vi "data_waypoint_ref.vi"() -> ()   [LabVIEW 2018] (continued)
"Y"=530209.4196220397}, {"X"=175331.62295978758, "Y"=530209.4709902672}, {"X"=175331.66061267612, "Y"=530209.5217040731}, {"X"=175331.69814321943, "Y"=530209.5723827237}, {"X"=175331.73536540987, "Y"=530209.6233275409}, {"X"=175331.77258882776, "Y"=530209.6746885533}, {"X"=175331.80997591818, "Y"=530209.7262832607}, {"X"=175331.8481199299, "Y"=530209.7774340136}, {"X"=175331.88623244286, "Y"=530209.8287158216}, {"X"=175331.9241847472, "Y"=530209.8794387324}, {"X"=175331.96143662307, "Y"=530209.9299384085}, {"X"=175331.99790744064, "Y"=530209.9799065489}, {"X"=175332.03363035072, "Y"=530210.0303718917}, {"X"=175332.07052518567, "Y"=530210.0802477727}, {"X"=175332.10833857156, "Y"=530210.1304217139}, {"X"=175332.14653489395, "Y"=530210.1818897336}, {"X"=175332.1846024039, "Y"=530210.2341328121}, {"X"=175332.22300738035, "Y"=530210.2869697822}, {"X"=175332.2621362657, "Y"=530210.339582644}, {"X"=175332.30199405577, "Y"=530210.3918626182}, {"X"=175332.34141600237, "Y"=530210.4441305593}, {"X"=175332.38041804795, "Y"=530210.4963853122}, {"X"=175332.4185211116, "Y"=530210.5486704636}, {"X"=175332.45682697443, "Y"=530210.5997386106}, {"X"=175332.49514308042, "Y"=530210.6506768743}, {"X"=175332.53412157384, "Y"=530210.7006542655}, {"X"=175332.57272378285, "Y"=530210.7512909137}, {"X"=175332.61101197888, "Y"=530210.8029773051}, {"X"=175332.64921056182, "Y"=530210.8558148851}, {"X"=175332.68851538797, "Y"=530210.9095182215}, {"X"=175332.72771294997, "Y"=530210.9640942254}, {"X"=175332.76750234602, "Y"=530211.0190136484}, {"X"=175332.80752506072, "Y"=530211.0731554804}, {"X"=175332.84765670967, "Y"=530211.1269895624}, {"X"=175332.88795444716, "Y"=530211.1803758806}, {"X"=175332.92839109115, "Y"=530211.234007068}, {"X"=175332.96848531367, "Y"=530211.2886669956}, {"X"=175333.0089040344, "Y"=530211.3437299544}, {"X"=175333.0491415058, "Y"=530211.3989066537}, {"X"=175333.08910233053, "Y"=530211.4539887221}, {"X"=175333.1285585995, "Y"=530211.5088869324}, {"X"=175333.16815412405, "Y"=530211.5626471259}, {"X"=175333.20753422027, "Y"=530211.6163446938}, {"X"=175333.2473421582, "Y"=530211.6697457767}, {"X"=175333.28705198405, "Y"=530211.724119386}, {"X"=175333.3265540142, "Y"=530211.779216127}, {"X"=175333.3660775373, "Y"=530211.8349931492}, {"X"=175333.40622949848, "Y"=530211.8900102822}, {"X"=175333.44650034822, "Y"=530211.9444932247}, {"X"=175333.48723672854, "Y"=530211.9985430562}, {"X"=175333.52736064664, "Y"=530212.0530630564}, {"X"=175333.56740341955, "Y"=530212.1080017141}, {"X"=175333.6077093309, "Y"=530212.1626599086}, {"X"=175333.64857199727, "Y"=530212.2168813988}, {"X"=175333.68922026566, "Y"=530212.2707905404}, {"X"=175333.72890749428, "Y"=530212.3247113958}, {"X"=175333.76778450757, "Y"=530212.3784270975}, {"X"=175333.80736747183, "Y"=530212.4321351693}, {"X"=175333.84828877196, "Y"=530212.4858159842}, {"X"=175333.88984022452, "Y"=530212.539917797}, {"X"=175333.93109660895, "Y"=530212.5948872815}, {"X"=175333.97284515807, "Y"=530212.6497432184}, {"X"=175334.0142686215, "Y"=530212.7046001133}, {"X"=175334.05544437704, "Y"=530212.7586608616}, {"X"=175334.0959890387, "Y"=530212.8128810698}, {"X"=175334.13627522383, "Y"=530212.8671608662}, {"X"=175334.17651603464, "Y"=530212.9222742985}, {"X"=175334.2177644458, "Y"=530212.9772438075}, {"X"=175334.25957639978, "Y"=530213.0322760266}, {"X"=175334.30213095952, "Y"=530213.0865147257}, {"X"=175334.34455506905, "Y"=530213.1406738986}, {"X"=175334.38594238626, "Y"=530213.195288953}, {"X"=175334.42704816477, "Y"=530213.2499525625}, {"X"=175334.46824282644, "Y"=530213.3047191269}, {"X"=175334.50961381703, "Y"=530213.3595051488}, {"X"=175334.55108627415, "Y"=530213.4141565791}, {"X"=175334.59266786097, "Y"=530213.4679675244}, {"X"=175334.63399788298, "Y"=530213.5211776675}, {"X"=175334.6750819692, "Y"=530213.573293105}, {"X"=175334.71570326976, "Y"=530213.6252711763}, {"X"=175334.75589895574, "Y"=530213.6780007676}, {"X"=175334.79658751158, "Y"=530213.7311584209}, {"X"=175334.83711118187, "Y"=530213.7854730334}, {"X"=175334.87751620755, "Y"=530213.8401054167}, {"X"=175334.9179042401, "Y"=530213.894081924}, {"X"=175334.95911596806, "Y"=530213.9465288344}, {"X"=175334.99991220928, "Y"=530213.9986573323}, {"X"=175335.04026648914, "Y"=530214.050201127}, {"X"=175335.08012203232, "Y"=530214.1026320615}, {"X"=175335.12058568108, "Y"=530214.1555184657}, {"X"=175335.16164489972, "Y"=530214.2088137578}, {"X"=175335.2026623043, "Y"=530214.2629493396}, {"X"=175335.24292566493, "Y"=530214.317904002}, {"X"=175335.2838600399, "Y"=530214.3724194007}, {"X"=175335.32589039847, "Y"=530214.4264254693}, {"X"=175335.36913003057, "Y"=530214.4801915719}, {"X"=175335.4125249086, "Y"=530214.5343367882}, {"X"=175335.45555095756, "Y"=530214.5889669928}, {"X"=175335.49830331592, "Y"=530214.6433027806}, {"X"=175335.54073540578, "Y"=530214.6974685959}, {"X"=175335.58196774634, "Y"=530214.7521007617}, {"X"=175335.62354322325, "Y"=530214.8059483555}, {"X"=175335.66565024323, "Y"=530214.8586179304}, {"X"=175335.70747625933, "Y"=530214.9106157594}, {"X"=175335.7480881228, "Y"=530214.963002292}, {"X"=175335.7885573149, "Y"=530215.0144669515}, {"X"=175335.82880391076, "Y"=530215.0658434787}, {"X"=175335.86905572907, "Y"=530215.1162866012}, {"X"=175335.909482951, "Y"=530215.1667380838}, {"X"=175335.95024341732, "Y"=530215.2175526178}, {"X"=175335.9909282017, "Y"=530215.2700366036}, {"X"=175336.03225353497, "Y"=530215.3231646375}, {"X"=175336.0742294917, "Y"=530215.3758479197}, {"X"=175336.1162228887, "Y"=530215.4281371495}, {"X"=175336.15780792251, "Y"=530215.480420926}, {"X"=175336.198753351, "Y"=530215.5338830402}, {"X"=175336.2400447598, "Y"=530215.5884240265}, {"X"=175336.28280096015, "Y"=530215.6431649067}, {"X"=175336.32627274963, "Y"=530215.697862611}, {"X"=175336.3695396637, "Y"=530215.7518728063}, {"X"=175336.41189431006, "Y"=530215.8050133444}, {"X"=175336.4530581296, "Y"=530215.857140764}, {"X"=175336.4923324384, "Y"=530215.9083226097}, {"X"=175336.53024073623, "Y"=530215.9582587824}, {"X"=175336.56758054454, "Y"=530216.0079569012}, {"X"=175336.60624975662, "Y"=530216.0567010613}, {"X"=175336.64522401133, "Y"=530216.1052567544}, {"X"=175336.68329837156, "Y"=530216.1538350807}, {"X"=175336.72042406868, "Y"=530216.2021165418}, {"X"=175336.75789178454, "Y"=530216.2498342964}, {"X"=175336.79601195845, "Y"=530216.2977277045}, {"X"=175336.83490120104, "Y"=530216.3474945049}, {"X"=175336.8747391946, "Y"=530216.3987878956}, {"X"=175336.9155644031, "Y"=530216.4511349584}, {"X"=175336.9565872925, "Y"=530216.5038343738}, {"X"=175336.99702923294, "Y"=530216.5562757964}, {"X"=175337.03653662247, "Y"=530216.608701107}, {"X"=175337.07562676386, "Y"=530216.6599112444}, {"X"=175337.11431845836, "Y"=530216.7105731766}, {"X"=175337.15316399393, "Y"=530216.7608384356}, {"X"=175337.19213873718, "Y"=530216.8122653349}, {"X"=175337.232309873, "Y"=530216.8641903627}, {"X"=175337.27302243776, "Y"=530216.9167896998}, {"X"=175337.31390302093, "Y"=530216.9698935254}, {"X"=175337.3542175054, "Y"=530217.0235705986}, {"X"=175337.39383505605, "Y"=530217.0782097556}, {"X"=175337.43345427106, "Y"=530217.1331130541}, {"X"=175337.4731671136, "Y"=530217.1885266124}, {"X"=175337.51269825146, "Y"=530217.2435999815}, {"X"=175337.55194491986, "Y"=530217.2977274793}, {"X"=175337.59038441366, "Y"=530217.3505776902}, {"X"=175337.62842923752, "Y"=530217.40235916}, {"X"=175337.6661001939, "Y"=530217.4535179922}, {"X"=175337.70416076016, "Y"=530217.5037300759}, {"X"=175337.7420038972, "Y"=530217.5544022826}, {"X"=175337.7794317696, "Y"=530217.6051323175}, {"X"=175337.81701866104, "Y"=530217.6563202547}, {"X"=175337.8544032769, "Y"=530217.708001567}, {"X"=175337.8925377935, "Y"=530217.7595608027}, {"X"=175337.93128742423, "Y"=530217.8109495258}, {"X"=175337.9695507337, "Y"=530217.8629301275}, {"X"=175338.0082516581, "Y"=530217.9152235296}, {"X"=175338.04761985684, "Y"=530217.967611521}, {"X"=175338.08728319546, "Y"=530218.0209597816}, {"X"=175338.1271335317, "Y"=530218.0749423284}, {"X"=175338.16702309356, "Y"=530218.1290091096}, {"X"=175338.20661768012, "Y"=530218.1830734315}, {"X"=175338.2461740608, "Y"=530218.2367982493}, {"X"=175338.28507050654, "Y"=530218.2905139152}, {"X"=175338.32402685797, "Y"=530218.3435179845}, {"X"=175338.3628983841, "Y"=530218.3962936742}, {"X"=175338.40248170623, "Y"=530218.4477409829}, {"X"=175338.44199884526, "Y"=530218.4989731741}, {"X"=175338.4810465143, "Y"=530218.5499037582}, {"X"=175338.51934318643, "Y"=530218.600885391}, {"X"=175338.55710943416, "Y"=530218.6522204147}, {"X"=175338.5948762553, "Y"=530218.7037507715}, {"X"=175338.6338252904, "Y"=530218.7548769822}, {"X"=175338.6739002579, "Y"=530218.8060364973}, {"X"=175338.71384854216, "Y"=530218.8583928163}, {"X"=175338.753222827, "Y"=530218.9113457106}, {"X"=175338.792356318, "Y"=530218.9646467023}, {"X"=175338.8311580059, "Y"=530219.01837153}, {"X"=175338.87071642242, "Y"=530219.0715880294}, {"X"=175338.91075334582, "Y"=530219.1254668134}, {"X"=175338.95190623117, "Y"=530219.1793034604}, {"X"=175338.99320496703, "Y"=530219.2336380056}, {"X"=175339.03450596903, "Y"=530219.2878393602}, {"X"=175339.07593600373, "Y"=530219.3419426669}, {"X"=175339.1173234146, "Y"=530219.3954090409}, {"X"=175339.15756587937, "Y"=530219.4490019855}, {"X"=175339.196607049, "Y"=530219.5022366615}, {"X"=175339.23502417348, "Y"=530219.5550181346}, {"X"=175339.27417272714, "Y"=530219.6071215451}, {"X"=175339.31415161595, "Y"=530219.6584433867}, {"X"=175339.35397403524, "Y"=530219.7095736838}, {"X"=175339.3928394618, "Y"=530219.7608854916}, {"X"=175339.43153280398, "Y"=530219.8121156775}, {"X"=175339.4711378264, "Y"=530219.8631167639}, {"X"=175339.5113195704, "Y"=530219.9153447627}, {"X"=175339.5514793716, "Y"=530219.968542844}, {"X"=175339.59169131416, "Y"=530220.0223001395}, {"X"=175339.63130955625, "Y"=530220.077183476}, {"X"=175339.6713096225, "Y"=530220.1317837801}, {"X"=175339.71162398445, "Y"=530220.1860302234}, {"X"=175339.75238126508, "Y"=530220.2396849147}, {"X"=175339.79291413393, "Y"=530220.2938363759}, {"X"=175339.8341795131, "Y"=530220.3476771363}, {"X"=175339.87538622756, "Y"=530220.4017489201}, {"X"=175339.91570330068, "Y"=530220.4557134501}, {"X"=175339.95501255686, "Y"=530220.5094489943}, {"X"=175339.99378179503, "Y"=530220.5623881428}, {"X"=175340.032220397, "Y"=530220.614045269}, {"X"=175340.0706813909, "Y"=530220.6642850373}, {"X"=175340.1095277134, "Y"=530220.7136280148}, {"X"=175340.1483784491, "Y"=530220.7632662015}, {"X"=175340.1866975091, "Y"=530220.8131345876}, {"X"=175340.22491300027, "Y"=530220.8627269252}, {"X"=175340.26314188118, "Y"=530220.9126532906}, {"X"=175340.30124549245, "Y"=530220.9624546103}, {"X"=175340.3389347308, "Y"=530221.0126145277}, {"X"=175340.3772862895, "Y"=530221.0623907007}, {"X"=175340.41577064258, "Y"=530221.1127436082}, {"X"=175340.45473172294, "Y"=530221.1634558148}, {"X"=175340.49399150687, "Y"=530221.2139340698}, {"X"=175340.53319028806, "Y"=530221.2641516883}, {"X"=175340.57132779274, "Y"=530221.3143324822}, {"X"=175340.60874069866, "Y"=530221.3645043136}, {"X"=175340.64630832113, "Y"=530221.4133749353}, {"X"=175340.68330462027, "Y"=530221.4616479168}, {"X"=175340.7200604363, "Y"=530221.5097728887}, {"X"=175340.7568127796, "Y"=530221.5576215149}, {"X"=175340.79352235922, "Y"=530221.6056866894}, {"X"=175340.83133687428, "Y"=530221.6532746962}, {"X"=175340.86972653927, "Y"=530221.701257226}, {"X"=175340.9080893437, "Y"=530221.7497437114}, {"X"=175340.9458108464, "Y"=530221.7991321841}, {"X"=175340.98414187023, "Y"=530221.8497574623}, {"X"=175341.02349582317, "Y"=530221.9009324348}, {"X"=175341.06375182403, "Y"=530221.9531158272}, {"X"=175341.1044829561, "Y"=530222.005719567}, {"X"=175341.14595957266, "Y"=530222.0579060195}, {"X"=175341.1872804957, "Y"=530222.1101617429}, {"X"=175341.2283713614, "Y"=530222.1619009508}, {"X"=175341.26824615517, "Y"=530222.213376271}, {"X"=175341.3077069612, "Y"=530222.2638406174}, {"X"=175341.3464592256, "Y"=530222.3143336911}, {"X"=175341.38514233282, "Y"=530222.3636039045}, {"X"=175341.42348113446, "Y"=530222.4123623798}, {"X"=175341.4619506573, "Y"=530222.4606942837}, {"X"=175341.500862789, "Y"=530222.5080282264}, {"X"=175341.53989545174, "Y"=530222.5556858942}, {"X"=175341.57855971582, "Y"=530222.6045743736}, {"X"=175341.61733350207, "Y"=530222.6548576218}, {"X"=175341.65613315726, "Y"=530222.7061030421}, {"X"=175341.69501567204, "Y"=530222.7578132504}, {"X"=175341.7343073941, "Y"=530222.8095144829}, {"X"=175341.77426430586, "Y"=530222.8600028963}, {"X"=175341.81392813384, "Y"=530222.9102291381}, {"X"=175341.85343851932, "Y"=530222.9594858147}, {"X"=175341.89225202618, "Y"=530223.0088222381}, {"X"=175341.93099129558, "Y"=530223.0579147108}, {"X"=175341.96965254052, "Y"=530223.1075823216}, {"X"=175342.0079390977, "Y"=530223.1578514714}, {"X"=175342.04531629087, "Y"=530223.208234289}, {"X"=175342.0823620307, "Y"=530223.2582584881}, {"X"=175342.12036757922, "Y"=530223.3069524673}, {"X"=175342.15868380744, "Y"=530223.3555689492}, {"X"=175342.19669862968, "Y"=530223.4053061692}, {"X"=175342.235050533, "Y"=530223.455206654}, {"X"=175342.2738534825, "Y"=530223.5063710476}, {"X"=175342.31314116152, "Y"=530223.5582054758}, {"X"=175342.35286638304, "Y"=530223.6106301709}, {"X"=175342.39277461008, "Y"=530223.6626336892}, {"X"=175342.43220801378, "Y"=530223.7146241793}, {"X"=175342.47159401196, "Y"=530223.7661575475}, {"X"=175342.51108410227, "Y"=530223.8175463284}, {"X"=175342.55094774097, "Y"=530223.869450092}, {"X"=175342.5912302505, "Y"=530223.9216189857}, {"X"=175342.63127412286, "Y"=530223.9742658229}, {"X"=175342.67080800404, "Y"=530224.0272881878}, {"X"=175342.71031867288, "Y"=530224.0796480348}, {"X"=175342.74951846778, "Y"=530224.1317202356}, {"X"=175342.78877232302, "Y"=530224.1828999498}, {"X"=175342.82772654106, "Y"=530224.2342991909}, {"X"=175342.86694903608, "Y"=530224.2847575897}, {"X"=175342.90560732182, "Y"=530224.3358291847}, {"X"=175342.94384633898, "Y"=530224.3871017921}, {"X"=175342.9820561291, "Y"=530224.4380759329}, {"X"=175343.02040845525, "Y"=530224.4887244644}, {"X"=175343.05860425235, "Y"=530224.539158146}, {"X"=175343.09711823752, "Y"=530224.5899571424}, {"X"=175343.1359562095, "Y"=530224.6415875782}, {"X"=175343.17549843973, "Y"=530224.6935377966}, {"X"=175343.21551242692, "Y"=530224.7456653102}, {"X"=175343.25560978387, "Y"=530224.7972276604}, {"X"=175343.29504013137, "Y"=530224.849386863}, {"X"=175343.3341498303, "Y"=530224.9012462393}, {"X"=175343.37274251977, "Y"=530224.9538052416}, {"X"=175343.41201237464, "Y"=530225.0068095207}, {"X"=175343.451815017, "Y"=530225.0602606118}, {"X"=175343.49195184934, "Y"=530225.1131957419}, {"X"=175343.53112082684, "Y"=530225.1662347257}, {"X"=175343.56961757506, "Y"=530225.219001554}, {"X"=175343.6080597585, "Y"=530225.2706864333}, {"X"=175343.64636462432, "Y"=530225.3217635131}, {"X"=175343.68403406208, "Y"=530225.3727314826}, {"X"=175343.7218600944, "Y"=530225.4236357275}, {"X"=175343.7595005975, "Y"=530225.4756059833}, {"X"=175343.79804115012, "Y"=530225.5279087643}, {"X"=175343.8375512105, "Y"=530225.5809689405}, {"X"=175343.87768913654, "Y"=530225.634275872}, {"X"=175343.917179842, "Y"=530225.6888821401}, {"X"=175343.95703650004, "Y"=530225.7435317221}, {"X"=175343.99699233004, "Y"=530225.7993696701}, {"X"=175344.0379195635, "Y"=530225.8560071833}, {"X"=175344.07954486008, "Y"=530225.9129678269}, {"X"=175344.1215070291, "Y"=530225.9700218146}, {"X"=175344.16306955542, "Y"=530226.0270237095}, {"X"=175344.20444305483, "Y"=530226.0836044145}, {"X"=175344.2454281164, "Y"=530226.140028664}, {"X"=175344.2863313288, "Y"=530226.1963310726}, {"X"=175344.32693259235, "Y"=530226.2520683417}, {"X"=175344.3668732474, "Y"=530226.3081693741}, {"X"=175344.40610914843, "Y"=530226.3646831337}, {"X"=175344.44565920217, "Y"=530226.4204934239}, {"X"=175344.48556397823, "Y"=530226.4755424161}, {"X"=175344.52579878274, "Y"=530226.5292641538}, {"X"=175344.56470778922, "Y"=530226.5830608321}, {"X"=175344.60305079306, "Y"=530226.6368625081}, {"X"=175344.64138657736, "Y"=530226.6909194754}, {"X"=175344.6803523717, "Y"=530226.7450500538}, {"X"=175344.7192578378, "Y"=530226.8000498302}, {"X"=175344.75917082647, "Y"=530226.8551809292}, {"X"=175344.79916464357, "Y"=530226.9115892368}, {"X"=175344.83981818473, "Y"=530226.9691365355}, {"X"=175344.88087487346, "Y"=530227.0279256878}, {"X"=175344.92272513863, "Y"=530227.0869855267}, {"X"=175344.96484817393, "Y"=530227.1460290228}, {"X"=175345.00702341314, "Y"=530227.2047527262}, {"X"=175345.04837276042, "Y"=530227.2636608795}, {"X"=175345.08951531787, "Y"=530227.322132361}, {"X"=175345.13091765594, "Y"=530227.3797862194}, {"X"=175345.17261180005, "Y"=530227.4369697464}, {"X"=175345.2138841165, "Y"=530227.4943875886}, {"X"=175345.25474182, "Y"=530227.5523837806}, {"X"=175345.2953319248, "Y"=530227.6103496855}, {"X"=175345.33608077082, "Y"=530227.6677768407}, {"X"=175345.3767031518, "Y"=530227.7246727465}, {"X"=175345.41711203125, "Y"=530227.7815592935}, {"X"=175345.45734774778, "Y"=530227.8385984013}, {"X"=175345.49814907316, "Y"=530227.8961008744}, {"X"=175345.53987397553, "Y"=530227.9535040656}, {"X"=175345.58270584818, "Y"=530228.0105188708}, {"X"=175345.62524984934, "Y"=530228.0681371794}, {"X"=175345.66747818922, "Y"=530228.1265477482}, {"X"=175345.70959393718, "Y"=530228.1852261261}, {"X"=175345.7526580195, "Y"=530228.2440892733}, {"X"=175345.79605483665, "Y"=530228.3031445545}, {"X"=175345.8397833751, "Y"=530228.362049028}, {"X"=175345.8829142793, "Y"=530228.4219463692}, {"X"=175345.92626609065, "Y"=530228.4816599311}, {"X"=175345.96973678764, "Y"=530228.5405385285}, {"X"=175346.0128790672, "Y"=530228.5985868099}, {"X"=175346.05557086875, "Y"=530228.6564643917}, {"X"=175346.09855932498, "Y"=530228.7140148013}, {"X"=175346.14169494555, "Y"=530228.7716069507}, {"X"=175346.18538720495, "Y"=530228.8284227776}, {"X"=175346.2289090404, "Y"=530228.8851192427}, {"X"=175346.27231195508, "Y"=530228.9411379342}, {"X"=175346.31467855422, "Y"=530228.9977745438}, {"X"=175346.3565197893, "Y"=530229.0540797464}, {"X"=175346.398209656, "Y"=530229.1098182551}, {"X"=175346.44036334916, "Y"=530229.1648461967}, {"X"=175346.48222626268, "Y"=530229.2206929632}, {"X"=175346.5240881895, "Y"=530229.2768060985}, {"X"=175346.56605635298, "Y"=530229.3332008257}, {"X"=175346.60913138627, "Y"=530229.3894735328}, {"X"=175346.65260054462, "Y"=530229.4460303147}, {"X"=175346.6961474528, "Y"=530229.5031207076}, {"X"=175346.73861139643, "Y"=530229.5606304918}, {"X"=175346.78057418144, "Y"=530229.6182061245}, {"X"=175346.8221392308, "Y"=530229.6754743905}, {"X"=175346.8638107502, "Y"=530229.7325026138}, {"X"=175346.90517967637, "Y"=530229.789648263}, {"X"=175346.94734387382, "Y"=530229.8467382959}, {"X"=175346.99017519283, "Y"=530229.9032714318}, {"X"=175347.03319368736, "Y"=530229.9604987887}, {"X"=175347.07558367634, "Y"=530230.0181630625}, {"X"=175347.1179610232, "Y"=530230.0760460165}, {"X"=175347.16041506414, "Y"=530230.1341029915}, {"X"=175347.20272800326, "Y"=530230.1926742499}, {"X"=175347.24512683423, "Y"=530230.2515349273}, {"X"=175347.2874182252, "Y"=530230.3109086764}, {"X"=175347.3299874161, "Y"=530230.3695679661}, {"X"=175347.37305761402, "Y"=530230.4275088108}, {"X"=175347.41586943413, "Y"=530230.4849409934}, {"X"=175347.45826517747, "Y"=530230.5418549861}, {"X"=175347.50003243302, "Y"=530230.5983091341}, {"X"=175347.54152667837, "Y"=530230.6550004845}, {"X"=175347.5828384125, "Y"=530230.7116779468}, {"X"=175347.62513317316, "Y"=530230.7676899249}, {"X"=175347.66725613666, "Y"=530230.8237168362}, {"X"=175347.70895552073, "Y"=530230.8796850655}, {"X"=175347.75047259853, "Y"=530230.936010097}, {"X"=175347.79224858, "Y"=530230.992420933}, {"X"=175347.83379821095, "Y"=530231.0501731497}, {"X"=175347.87598747012, "Y"=530231.1085583183}, {"X"=175347.91865063147, "Y"=530231.1672461922}, {"X"=175347.96190239483, "Y"=530231.2254839465}, {"X"=175348.0049063384, "Y"=530231.2837890219}, {"X"=175348.04776506487, "Y"=530231.3412110822}, {"X"=175348.09002578325, "Y"=530231.3988968299}, {"X"=175348.1320544484, "Y"=530231.4565921396}, {"X"=175348.17388105046, "Y"=530231.5145510836}, {"X"=175348.2155488722, "Y"=530231.5718334815}, {"X"=175348.25715479362, "Y"=530231.6288519169}, {"X"=175348.298702659, "Y"=530231.6857062625}, {"X"=175348.34000642208, "Y"=530231.7423881912}, {"X"=175348.38131569765, "Y"=530231.7988370324}, {"X"=175348.42291422226, "Y"=530231.8557500527}, {"X"=175348.4651085602, "Y"=530231.9128555425}, {"X"=175348.5074611014, "Y"=530231.9701425808}, {"X"=175348.54977016072, "Y"=530232.0277038846}, {"X"=175348.59204602803, "Y"=530232.085123225}, {"X"=175348.63413675412, "Y"=530232.1425386709}, {"X"=175348.6759034338, "Y"=530232.200305787}, {"X"=175348.71787818449, "Y"=530232.2589446416}, {"X"=175348.76045198838, "Y"=530232.317371966}, {"X"=175348.80372661783, "Y"=530232.3755574945}, {"X"=175348.8467706997, "Y"=530232.4330600277}, {"X"=175348.88973412907, "Y"=530232.4902464917}, {"X"=175348.9325830176, "Y"=530232.5467385219}, {"X"=175348.97525145314, "Y"=530232.6036150943}, {"X"=175349.01743876605, "Y"=530232.6613454565}, {"X"=175349.05979153828, "Y"=530232.719614725}, {"X"=175349.1024098835, "Y"=530232.7775280537}, {"X"=175349.1453880101, "Y"=530232.8351950453}, {"X"=175349.18802687485, "Y"=530232.8922581619}, {"X"=175349.23083361104, "Y"=530232.9488757306}, {"X"=175349.2737960797, "Y"=530233.0057381197}, {"X"=175349.31699101478, "Y"=530233.0627330062}, {"X"=175349.35974836414, "Y"=530233.1203262894}, {"X"=175349.40281906206, "Y"=530233.1778453963}, {"X"=175349.44570093186, "Y"=530233.2353117875}, {"X"=175349.4887297444, "Y"=530233.2927455591}, {"X"=175349.53150355406, "Y"=530233.3505141508}, {"X"=175349.5747305128, "Y"=530233.4081582131}, {"X"=175349.61876782076, "Y"=530233.4660540435}, {"X"=175349.66334610982, "Y"=530233.5235709278}, {"X"=175349.70725425257, "Y"=530233.5815204117}, {"X"=175349.7504956164, "Y"=530233.639544004}, {"X"=175349.79353860093, "Y"=530233.6972796193}, {"X"=175349.83754390068, "Y"=530233.7539336112}, {"X"=175349.88171600256, "Y"=530233.8106814525}, {"X"=175349.92563081637, "Y"=530233.8675898704}, {"X"=175349.96906826223, "Y"=530233.9251234373}, {"X"=175350.01293208322, "Y"=530233.9821629709}, {"X"=175350.05650620023, "Y"=530234.0394841522}, {"X"=175350.09989550654, "Y"=530234.096613872}, {"X"=175350.14314725774, "Y"=530234.1536552103}, {"X"=175350.18660337463, "Y"=530234.2106127074}, {"X"=175350.2305396156, "Y"=530234.2675798872}, {"X"=175350.2749188809, "Y"=530234.3239919407}, {"X"=175350.31926038675, "Y"=530234.3805162015}, {"X"=175350.36325309795, "Y"=530234.4371080835}, {"X"=175350.40650135832, "Y"=530234.4938686392}, {"X"=175350.44973874703, "Y"=530234.5505470965}, {"X"=175350.49322314374, "Y"=530234.6074834237}, {"X"=175350.5372465261, "Y"=530234.6645657729}, {"X"=175350.58161553548, "Y"=530234.7214062652}, {"X"=175350.62636864078, "Y"=530234.7781335282}, {"X"=175350.67098936674, "Y"=530234.8347268899}, {"X"=175350.71522448817, "Y"=530234.8915222726}, {"X"=175350.75861984972, "Y"=530234.9483045933}, {"X"=175350.80163544806, "Y"=530235.0051679431}, {"X"=175350.8455027871, "Y"=530235.061300714}, {"X"=175350.88993979365, "Y"=530235.1168702191}, {"X"=175350.93419405032, "Y"=530235.1720451514}, {"X"=175350.97797018028, "Y"=530235.2272858657}, {"X"=175351.0211706906, "Y"=530235.2819733487}, {"X"=175351.06420086315, "Y"=530235.3368710969}, {"X"=175351.1069546017, "Y"=530235.391745242}, {"X"=175351.14969397328, "Y"=530235.4471543846}, {"X"=175351.19290508452, "Y"=530235.5030349332}, {"X"=175351.23708086298, "Y"=530235.5592333905}, {"X"=175351.28094664667, "Y"=530235.6163428451}, {"X"=175351.32507018273, "Y"=530235.6737500923}, {"X"=175351.36946815113, "Y"=530235.7311032579}, {"X"=175351.4141272058, "Y"=530235.7883812926}, {"X"=175351.45875193508, "Y"=530235.845434128}, {"X"=175351.5033432786, "Y"=530235.9016790844}, {"X"=175351.5477972615, "Y"=530235.9573007046}, {"X"=175351.5920627689, "Y"=530236.0123890406}, {"X"=175351.63490704828, "Y"=530236.0676302855}, {"X"=175351.67720670445, "Y"=530236.1229175301}, {"X"=175351.71963278952, "Y"=530236.1781233831}, {"X"=175351.76294240737, "Y"=530236.2322667169}, {"X"=175351.80625901482, "Y"=530236.2860770716}, {"X"=175351.84902049394, "Y"=530236.3393729797}, {"X"=175351.89089530785, "Y"=530236.3929711628}, {"X"=175351.9331973055, "Y"=530236.4457479022}, {"X"=175351.97514771618, "Y"=530236.498248212}, {"X"=175352.01617310618, "Y"=530236.5512595625}, {"X"=175352.05664432573, "Y"=530236.6049850797}, {"X"=175352.09796583082, "Y"=530236.6580865675}, {"X"=175352.13995707338, "Y"=530236.7103159536}, {"X"=175352.18166292325, "Y"=530236.7621876963}, {"X"=175352.22252090828, "Y"=530236.813099689}, {"X"=175352.26255605364, "Y"=530236.8637288735}, {"X"=175352.30208352584, "Y"=530236.9137169486}, {"X"=175352.34150491114, "Y"=530236.9634744846}, {"X"=175352.38042420865, "Y"=530237.0135842154}, {"X"=175352.4199305173, "Y"=530237.0639053108}, {"X"=175352.45956587067, "Y"=530237.114131686}, {"X"=175352.49899166732, "Y"=530237.1641844318}, {"X"=175352.53829575534, "Y"=530237.2141165627}, {"X"=175352.5774806659, "Y"=530237.2632843519}, {"X"=175352.6156511215, "Y"=530237.3132742075}, {"X"=175352.6533883326, "Y"=530237.3629312733}, {"X"=175352.6910130333, "Y"=530237.4119815769}, {"X"=175352.72911552244, "Y"=530237.4611514483}, {"X"=175352.7674107072, "Y"=530237.5110854433}, {"X"=175352.80628102296, "Y"=530237.5626092828}, {"X"=175352.84566256969, "Y"=530237.6153813166}, {"X"=175352.886305737, "Y"=530237.6688455134}, {"X"=175352.92686425932, "Y"=530237.7224420327}, {"X"=175352.96628213656, "Y"=530237.776421486}, {"X"=175353.00479581486, "Y"=530237.8295612222}, {"X"=175353.04309125987, "Y"=530237.8813875283}, {"X"=175353.0805856114, "Y"=530237.9321951261}, {"X"=175353.1178263727, "Y"=530237.9820145867}, {"X"=175353.15486826623, "Y"=530238.031681473}, {"X"=175353.19223656916, "Y"=530238.0808956837}, {"X"=175353.22936573613, "Y"=530238.1307199139}, {"X"=175353.26626025818, "Y"=530238.1808755734}, {"X"=175353.3027933256, "Y"=530238.2313119823}, {"X"=175353.33960005036, "Y"=530238.2823335917}, {"X"=175353.37707444988, "Y"=530238.3338859645}, {"X"=175353.41547161504, "Y"=530238.386566564}, {"X"=175353.45446338505, "Y"=530238.4399313043}, {"X"=175353.49378934092, "Y"=530238.4939798436}, {"X"=175353.53226842728, "Y"=530238.5480086806}, {"X"=175353.57047974097, "Y"=530238.6019472994}, {"X"=175353.60875617847, "Y"=530238.6557414449}, {"X"=175353.6469764394, "Y"=530238.7094103412}, {"X"=175353.68457545002, "Y"=530238.7638723999}, {"X"=175353.72234228044, "Y"=530238.8184738057}, {"X"=175353.76045086328, "Y"=530238.8730198212}, {"X"=175353.79898426452, "Y"=530238.9271461678}, {"X"=175353.8375490814, "Y"=530238.9808107199}, {"X"=175353.8752460613, "Y"=530239.0342536401}, {"X"=175353.91189012938, "Y"=530239.0874910104}, {"X"=175353.94910051365, "Y"=530239.1393293964}, {"X"=175353.98627210603, "Y"=530239.1909281688}, {"X"=175354.02308637538, "Y"=530239.2430096754}, {"X"=175354.05967783305, "Y"=530239.2955291213}, {"X"=175354.09668178417, "Y"=530239.3488542204}, {"X"=175354.1341990515, "Y"=530239.4023320772}, {"X"=175354.17198692198, "Y"=530239.4562597376}, {"X"=175354.20951566947, "Y"=530239.5106276667}, {"X"=175354.24727854424, "Y"=530239.5653911263}, {"X"=175354.28528886437, "Y"=530239.6202604033}, {"X"=175354.3236916914, "Y"=530239.6751662572}, {"X"=175354.36217982642, "Y"=530239.7301650902}, {"X"=175354.401261916, "Y"=530239.784725996}, {"X"=175354.4399844256, "Y"=530239.8399039346}, {"X"=175354.47800392206, "Y"=530239.8951827234}, {"X"=175354.51573281956, "Y"=530239.9501405099}, {"X"=175354.55374814585, "Y"=530240.0043061222}, {"X"=175354.5920931261, "Y"=530240.0585195966}, {"X"=175354.6307848023, "Y"=530240.1125533618}, {"X"=175354.66938268108, "Y"=530240.1672211337}, {"X"=175354.70835670453, "Y"=530240.22178347}, {"X"=175354.74747454954, "Y"=530240.2767560309}, {"X"=175354.78668856682, "Y"=530240.3322011083}, {"X"=175354.82573295297, "Y"=530240.3880961786}, {"X"=175354.86442117963, "Y"=530240.4448679785}, {"X"=175354.90385480528, "Y"=530240.5017940709}, {"X"=175354.9438868584, "Y"=530240.5585985357}, {"X"=175354.98450460396, "Y"=530240.6151670938}, {"X"=175355.02560184867, "Y"=530240.6712336912}, {"X"=175355.0663030908, "Y"=530240.7269795968}, {"X"=175355.10590519384, "Y"=530240.7830661403}, {"X"=175355.1451417851, "Y"=530240.8386587655}, {"X"=175355.1843346686, "Y"=530240.8944490728}, {"X"=175355.22404374706, "Y"=530240.9501668296}, {"X"=175355.2643191493, "Y"=530241.0056886901}, {"X"=175355.30494895973, "Y"=530241.0609420296}, {"X"=175355.34536480953, "Y"=530241.1163314045}, {"X"=175355.38549545314, "Y"=530241.1717260601}, {"X"=175355.42590157175, "Y"=530241.2271199028}, {"X"=175355.466450924, "Y"=530241.2827253059}, {"X"=175355.50749417936, "Y"=530241.3382071704}, {"X"=175355.54871472975, "Y"=530241.3943377783}, {"X"=175355.5905385754, "Y"=530241.4498939218}, {"X"=175355.6317120192, "Y"=530241.5056695165}, {"X"=175355.6725872653, "Y"=530241.5612506543}, {"X"=175355.7131346146, "Y"=530241.6170791457}, {"X"=175355.7536999294, "Y"=530241.6726922737}, {"X"=175355.79431457655, "Y"=530241.7288135714}, {"X"=175355.83564892667, "Y"=530241.7844865855}, {"X"=175355.87750007684, "Y"=530241.8402923684}, {"X"=175355.9195047443, "Y"=530241.8958912657}, {"X"=175355.96087904507, "Y"=530241.9515952377}, {"X"=175356.0021839649, "Y"=530242.0072017458}, {"X"=175356.04336760036, "Y"=530242.0628308104}, {"X"=175356.08446281333, "Y"=530242.1185134072}, {"X"=175356.1253711881, "Y"=530242.1742165342}, {"X"=175356.16642529293, "Y"=530242.2294763982}, {"X"=175356.20768692662, "Y"=530242.2839210114}, {"X"=175356.24861907747, "Y"=530242.3386751397}, {"X"=175356.28909854963, "Y"=530242.3934161742}, {"X"=175356.3297216975, "Y"=530242.4482167154}, {"X"=175356.37073719004, "Y"=530242.5026975726}, {"X"=175356.4121149016, "Y"=530242.5571573845}, {"X"=175356.45343968744, "Y"=530242.6113920517}, {"X"=175356.4948522827, "Y"=530242.6656653044}, {"X"=175356.53583169985, "Y"=530242.7208310526}, {"X"=175356.57724413514, "Y"=530242.7765537826}, {"X"=175356.61908518994, "Y"=530242.8331442699}, {"X"=175356.66122786675, "Y"=530242.8895895861}, {"X"=175356.7031677672, "Y"=530242.9460588078}, {"X"=175356.74520092676, "Y"=530243.0017108984}, {"X"=175356.78699071577, "Y"=530243.0568376329}, {"X"=175356.82860514967, "Y"=530243.1110725575}, {"X"=175356.86955351502, "Y"=530243.1650197727}, {"X"=175356.90969446828, "Y"=530243.2182091132}, {"X"=175356.9490777895, "Y"=530243.2712996902}, {"X"=175356.98857629084, "Y"=530243.3234998218}, {"X"=175357.02793550797, "Y"=530243.375025569}, {"X"=175357.06710013995, "Y"=530243.4266473373}, {"X"=175357.10620575276, "Y"=530243.4780817132}, {"X"=175357.14540980468, "Y"=530243.5298554179}, {"X"=175357.18500684414, "Y"=530243.5818288475}, {"X"=175357.2246604417, "Y"=530243.6349596942}, {"X"=175357.2641467288, "Y"=530243.6890266448}, {"X"=175357.30388953027, "Y"=530243.7438730717}, {"X"=175357.34434687858, "Y"=530243.7989260455}, {"X"=175357.38561276108, "Y"=530243.853314052}, {"X"=175357.42714635562, "Y"=530243.9080741812}, {"X"=175357.46842059385, "Y"=530243.9631946698}, {"X"=175357.50957774406, "Y"=530244.0191612169}, {"X"=175357.55071779378, "Y"=530244.0753364675}, {"X"=175357.5918336218, "Y"=530244.1320090053}, {"X"=175357.63331725454, "Y"=530244.1881499484}, {"X"=175357.6750473695, "Y"=530244.2440715226}, {"X"=175357.7166139784, "Y"=530244.2995152301}, {"X"=175357.75781324354, "Y"=530244.3550454788}, {"X"=175357.79876509352, "Y"=530244.4101791265}, {"X"=175357.8395200305, "Y"=530244.4652223483}, {"X"=175357.88012770392, "Y"=530244.5204901953}, {"X"=175357.92098501846, "Y"=530244.5757073621}, {"X"=175357.96204256182, "Y"=530244.6303379341}, {"X"=175358.0031356214, "Y"=530244.6843968236}, {"X"=175358.04383856695, "Y"=530244.7389307731}, {"X"=175358.08452646548, "Y"=530244.7931695447}, {"X"=175358.12566475326, "Y"=530244.8472460592}, {"X"=175358.16694392514, "Y"=530244.9013388081}, {"X"=175358.20819046954, "Y"=530244.9557823667}, {"X"=175358.2494700914, "Y"=530245.0103279366}, {"X"=175358.29098381952, "Y"=530245.064361171}, {"X"=175358.33216177375, "Y"=530245.118073536}, {"X"=175358.3732513863, "Y"=530245.1718660723}, {"X"=175358.41425988183, "Y"=530245.2263869141}, {"X"=175358.45530746563, "Y"=530245.2806457151}, {"X"=175358.4961279473, "Y"=530245.3353901925}, {"X"=175358.53755439995, "Y"=530245.389565749}, {"X"=175358.57880946694, "Y"=530245.4429948742}, {"X"=175358.6194754227, "Y"=530245.4955001123}, {"X"=175358.65923557561, "Y"=530245.5475241211}, {"X"=175358.6986810228, "Y"=530245.5985601745}, {"X"=175358.73818095252, "Y"=530245.6497481184}, {"X"=175358.77788761366, "Y"=530245.7016557507}, {"X"=175358.81772277673, "Y"=530245.7538848643}, {"X"=175358.8581828618, "Y"=530245.8068668401}, {"X"=175358.89923729494, "Y"=530245.8601456174}, {"X"=175358.94051532645, "Y"=530245.9144559056}, {"X"=175358.9816894016, "Y"=530245.9692592768}, {"X"=175359.02267067126, "Y"=530246.024462766}, {"X"=175359.06317469152, "Y"=530246.0791293798}, {"X"=175359.10328494103, "Y"=530246.1330302408}, {"X"=175359.1426311365, "Y"=530246.1864572257}, {"X"=175359.18170182902, "Y"=530246.2389749364}, {"X"=175359.22067294916, "Y"=530246.2913686386}, {"X"=175359.26036426862, "Y"=530246.3431819814}, {"X"=175359.3002206982, "Y"=530246.3951147026}, {"X"=175359.33957727332, "Y"=530246.4472564398}, {"X"=175359.37847526275, "Y"=530246.4997835399}, {"X"=175359.41736539445, "Y"=530246.5517468553}, {"X"=175359.45611866727, "Y"=530246.6035596343}, {"X"=175359.49516651212, "Y"=530246.6552394703}, {"X"=175359.534532394, "Y"=530246.7066320259}, {"X"=175359.5738779074, "Y"=530246.7589269583}, {"X"=175359.61317105513, "Y"=530246.8120899559}, {"X"=175359.65284148513, "Y"=530246.8658334052}, {"X"=175359.6924238613, "Y"=530246.9197546942}, {"X"=175359.7321189642, "Y"=530246.9737555607}, {"X"=175359.7722131497, "Y"=530247.0267175318}, {"X"=175359.812302406, "Y"=530247.078607394}, {"X"=175359.8517182705, "Y"=530247.1301296569}, {"X"=175359.89077924602, "Y"=530247.180555317}, {"X"=175359.9290297936, "Y"=530247.2313018942}, {"X"=175359.96678072223, "Y"=530247.2823373973}, {"X"=175360.00470898786, "Y"=530247.3328329864}, {"X"=175360.04301417153, "Y"=530247.3831842932}, {"X"=175360.0812444498, "Y"=530247.4339664449}, {"X"=175360.11974357752, "Y"=530247.4852061785}, {"X"=175360.15889532102, "Y"=530247.5363762868}, {"X"=175360.19878413517, "Y"=530247.5878805108}, {"X"=175360.23892902656, "Y"=530247.6391142854}, {"X"=175360.278401387, "Y"=530247.6905731225}, {"X"=175360.31737113406, "Y"=530247.7419035878}, {"X"=175360.3562170554, "Y"=530247.7923964746}, {"X"=175360.39471564715, "Y"=530247.8425529867}, {"X"=175360.43373020628, "Y"=530247.8922584872}, {"X"=175360.47263689383, "Y"=530247.9426313309}, {"X"=175360.51171172748, "Y"=530247.9935541683}, {"X"=175360.55096069007, "Y"=530248.0452522838}, {"X"=175360.59049010673, "Y"=530248.0971371413}, {"X"=175360.63068016354, "Y"=530248.1486704462}, {"X"=175360.67107729564, "Y"=530248.2001354393}, {"X"=175360.71119287587, "Y"=530248.2510430022}, {"X"=175360.75040324742, "Y"=530248.3025725349}, {"X"=175360.78979999508, "Y"=530248.3545254847}, {"X"=175360.8304710297, "Y"=530248.4066589174}, {"X"=175360.87127768132, "Y"=530248.4591260182}, {"X"=175360.91191723972, "Y"=530248.5123017002}, {"X"=175360.9523743838, "Y"=530248.5657975603}, {"X"=175360.99262587648, "Y"=530248.618641429}, {"X"=175361.0330122471, "Y"=530248.6709654863}, {"X"=175361.0729788118, "Y"=530248.7224062232}, {"X"=175361.11191044463, "Y"=530248.7737323643}, {"X"=175361.1505965638, "Y"=530248.8241047515}, {"X"=175361.18968035345, "Y"=530248.8732595601}, {"X"=175361.22874977769, "Y"=530248.921748496}, {"X"=175361.26740235148, "Y"=530248.9697558712}, {"X"=175361.3060301731, "Y"=530249.0177799684}, {"X"=175361.34393528936, "Y"=530249.066737368}, {"X"=175361.38214647444, "Y"=530249.1170578811}, {"X"=175361.4216719192, "Y"=530249.1682002577}, {"X"=175361.46218246105, "Y"=530249.2199790122}, {"X"=175361.50222234274, "Y"=530249.2728556928}, {"X"=175361.54213471914, "Y"=530249.3257493963}, {"X"=175361.5823825225, "Y"=530249.3776443499}, {"X"=175361.62273221207, "Y"=530249.428344794}, {"X"=175361.6628429453, "Y"=530249.4785132093}, {"X"=175361.70243138418, "Y"=530249.528188167}, {"X"=175361.74098416534, "Y"=530249.578102579}, {"X"=175361.77956365625, "Y"=530249.6283642957}, {"X"=175361.81847626573, "Y"=530249.6783475681}, {"X"=175361.8581347175, "Y"=530249.7283353001}, {"X"=175361.8979152902, "Y"=530249.778284938}, {"X"=175361.93752073805, "Y"=530249.8283216615}, {"X"=175361.97688238163, "Y"=530249.8785866245}, {"X"=175362.0162104847, "Y"=530249.9285919806}, {"X"=175362.0553811717, "Y"=530249.978382486}, {"X"=175362.09459135542, "Y"=530250.0277489105}, {"X"=175362.1339222446, "Y"=530250.0774978804}, {"X"=175362.1736222086, "Y"=530250.1271469857}, {"X"=175362.21321350688, "Y"=530250.1768918592}, {"X"=175362.252683638, "Y"=530250.2270011243}, {"X"=175362.2924473459, "Y"=530250.2766389428}, {"X"=175362.33200780407, "Y"=530250.3264405108}, {"X"=175362.37099305278, "Y"=530250.376127239}, {"X"=175362.41009984864, "Y"=530250.4258801995}, {"X"=175362.44898119677, "Y"=530250.4751765631}, {"X"=175362.48782192072, "Y"=530250.52421334}, {"X"=175362.52699950442, "Y"=530250.5730404704}, {"X"=175362.5667985681, "Y"=530250.6220522263}, {"X"=175362.60660301094, "Y"=530250.6722892505}, {"X"=175362.64652048083, "Y"=530250.7230076215}, {"X"=175362.6858567776, "Y"=530250.7736921888}, {"X"=175362.7251310844, "Y"=530250.8240806081}, {"X"=175362.7639446701, "Y"=530250.8741296573}, {"X"=175362.8025109473, "Y"=530250.9235190699}, {"X"=175362.84085578495, "Y"=530250.9717071552}, {"X"=175362.87910314006, "Y"=530251.0198799929}, {"X"=175362.91751004552, "Y"=530251.0674885499}, {"X"=175362.95600635879, "Y"=530251.1153798591}, {"X"=175362.99435708468, "Y"=530251.1643636992}, {"X"=175363.0334184228, "Y"=530251.2137227969}, {"X"=175363.07259438004, "Y"=530251.2638029656}, {"X"=175363.11199823796, "Y"=530251.3139701424}, {"X"=175363.1513796253, "Y"=530251.364327171}, {"X"=175363.1906501197, "Y"=530251.4146268141}, {"X"=175363.22968945027, "Y"=530251.4646341368}, {"X"=175363.26866563145, "Y"=530251.5142531929}, {"X"=175363.3073697122, "Y"=530251.563214906}, {"X"=175363.34559084047, "Y"=530251.6127085537}, {"X"=175363.38380230192, "Y"=530251.6619292059}, {"X"=175363.42243679025, "Y"=530251.7104205436}, {"X"=175363.4610109799, "Y"=530251.7588898608}, {"X"=175363.49973307314, "Y"=530251.8073520857}, {"X"=175363.5383682305, "Y"=530251.8560709434}, {"X"=175363.57717002617, "Y"=530251.9048281554}, {"X"=175363.61560527026, "Y"=530251.9542412636}, {"X"=175363.65436447458, "Y"=530252.0032738473}, {"X"=175363.69337000587, "Y"=530252.0523334497}, {"X"=175363.7324087816, "Y"=530252.1018546579}, {"X"=175363.77137032332, "Y"=530252.1516169315}, {"X"=175363.81046026983, "Y"=530252.2025719273}, {"X"=175363.85010976103, "Y"=530252.253435373}, {"X"=175363.89048429485, "Y"=530252.3041590624}, {"X"=175363.9305881354, "Y"=530252.3547037531}, {"X"=175363.97065607106, "Y"=530252.4053872812}, {"X"=175364.0104260441, "Y"=530252.455955151}, {"X"=175364.05022246856, "Y"=530252.5055817852}, {"X"=175364.0895394326, "Y"=530252.5551210414}, {"X"=175364.12854528782, "Y"=530252.6042938508}, {"X"=175364.1669772529, "Y"=530252.6537979816}, {"X"=175364.2054922055, "Y"=530252.702908976}, {"X"=175364.24385568034, "Y"=530252.7514155437}, {"X"=175364.28218815473, "Y"=530252.799923314}, {"X"=175364.32078050665, "Y"=530252.848247191}, {"X"=175364.35987321084, "Y"=530252.8971334021}, {"X"=175364.39976063493, "Y"=530252.9472814032}, {"X"=175364.44051739766, "Y"=530252.9990649943}, {"X"=175364.48121062687, "Y"=530253.052132879}, {"X"=175364.5217449672, "Y"=530253.1050880281}, {"X"=175364.56172633727, "Y"=530253.1576607942}, {"X"=175364.60130530893, "Y"=530253.2095455242}, {"X"=175364.64039269785, "Y"=530253.2608368186}, {"X"=175364.67953891496, "Y"=530253.3116529188}, {"X"=175364.71831601113, 
